vi "Untitled 1.vi"() -> ()   [LabVIEW 2021]
uses:
  <vilib>/Instr/_visa.llb/VISA Configure Serial Port (Instr).vi
panel:
  out "x >= y?":bool
  out "x .and. y?":bool
  out "x < y?":bool
  out "Waveform Chart":dbl(graph)
  in  "STOP":bool
  out "Gauge":dbl(knob) scale=0.0..100.0
  out "0-100 Arası Manyetik Alan Değeri":string
  in  "Port Seçimi":refnum<visa-resource-name>
  # "CONTROLLING HALL EFFECT SENSOR WİTH ARDUİNO"
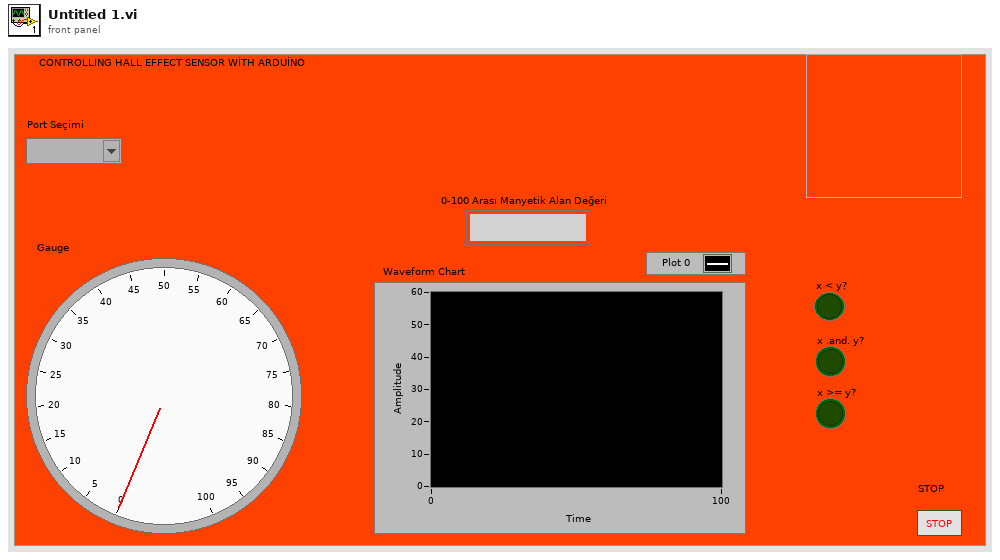
[diagram p1: front panel]
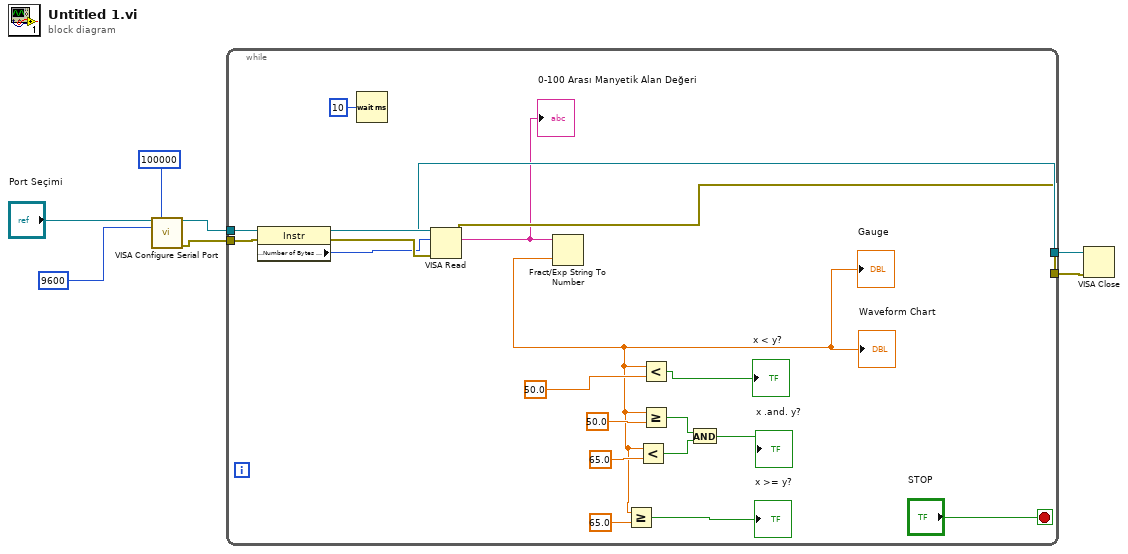
[diagram p0: block diagram]
diagram:
  n1 = call-poly "VISA Configure Serial Port"("VISA resource name"="Port Seçimi", "timeout (10sec)"=u32 100000, "baud rate (9600)"=u32 9600) -> ("VISA resource name out"=w4:refnum<visa-resource-name>, "error out"=w3:errorcluster)  [unwired: 11 in]
  n2 = while {
    tunnel: w4 -> [w27]
    tunnel: w3 -> [w26]
    tunnel: [w22] -> w2
    tunnel: [w21] -> w1
    stop <- "STOP" stop-if-true
    n3 = property class="Instr"(reference=w27, error in=w26) -> (reference out=w25:refnum<visa-resource-name>, error out=w24:errorcluster, "Serial Settings:Number of Bytes at Serial Port"=w23:u32)
    n4 = Wait (ms)(milliseconds to wait=u32 10) -> ()  [unwired: 1 out]
    n5 = VISA Read(VISA resource name=w25, byte count=w23, error in (no error)=w24) -> (VISA resource name out=w22:refnum<visa-resource-name>, read buffer=w20:string, error out=w21:errorcluster)  [unwired: 1 out]
    "0-100 Arası Manyetik Alan Değeri" <- w20
    n6 = Fract/Exp String To Number(string=w20) -> (number=w13:dbl)  [unwired: 3 in, 1 out]
    "Gauge" <- w13
    "Waveform Chart" <- w13
    n7 = Greater Or Equal?(x=w13, y=65.0) -> (x >= y?=→"x >= y?":bool)
    n8 = Less?(x=w13, y=65.0) -> (x < y?=w10:bool)
    n9 = Less?(x=w13, y=50.0) -> (x < y?=→"x < y?":bool)
    n10 = Greater Or Equal?(x=w13, y=50.0) -> (x >= y?=w11:bool)
    n11 = And(x=w11, y=w10) -> (x .and. y?=→"x .and. y?":bool)
  }
  n12 = VISA Close(VISA resource name=w2, error in (no error)=w1) -> ()  [unwired: 1 out]
